vi "Calc Arc Angles.vi"(9 "Position Scale":dbl=1.0, 10 "Arc CMD":T1={"N"=0.0, "GCODE"="", "X"=2.0396, "Y"=0.1665, "Z"=0.0, "E"=0.0, "I"=0.205, "J"=0.131, "S"=0.0, "F"=0.0, "Text"=""}, 11 "Initial CMD":T1={"N"=0.0, "GCODE"="", "X"=1.6296, "Y"=0.1665, "Z"=-0.05, "E"=0.0, "I"=0.0, "J"=0.0, "S"=0.0, "F"=0.0, "Text"=""}) -> (0 "travel angle out":dbl=114.84085989051317 format="%.5f", 2 "start angle (tangent)":dbl=212.57957005474344 format="%#_8g", 3 "R":dbl=0.2432817296880306 format="%#_9g")   [LabVIEW 2014]
uses:
  GCode Parser/GCode Command Cluster.ctl
panel:
  out "x*y":dbl=32.57957005474343
  out "V2Y":dbl=-0.13099999999999998
  out "V2X":dbl=0.20500000000000007
  out "V1Y":dbl=-0.13099999999999998
  out "V1X":dbl=-0.20500000000000007
  out "theta (degrees)":dbl=-114.84085989051317 format="%.2f"
  out "theta (radians)":dbl=-2.0043511209109495 format="%.3f"
  # "G01 X1.6296 Y0.1665 Z-0.0500\nG03 X2.0396 Y0.1665 I0.2050 J0.1310"
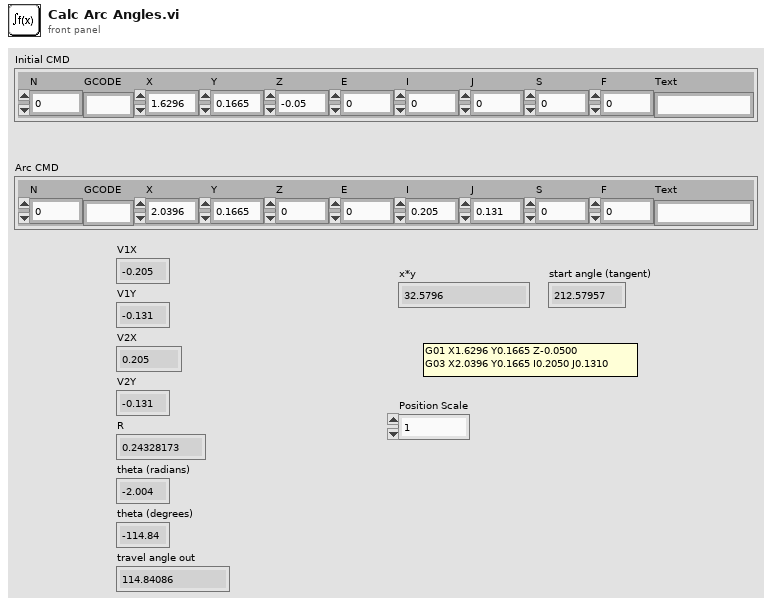
[diagram p1: front panel]
types:
  T1 = typedef "GCode Command Cluster.ctl" = cluster{"N":dbl, "GCODE":string, "X":dbl, "Y":dbl, "Z":dbl, "E":dbl, "I":dbl, "J":dbl, "S":dbl, "F":dbl, "Text":string}
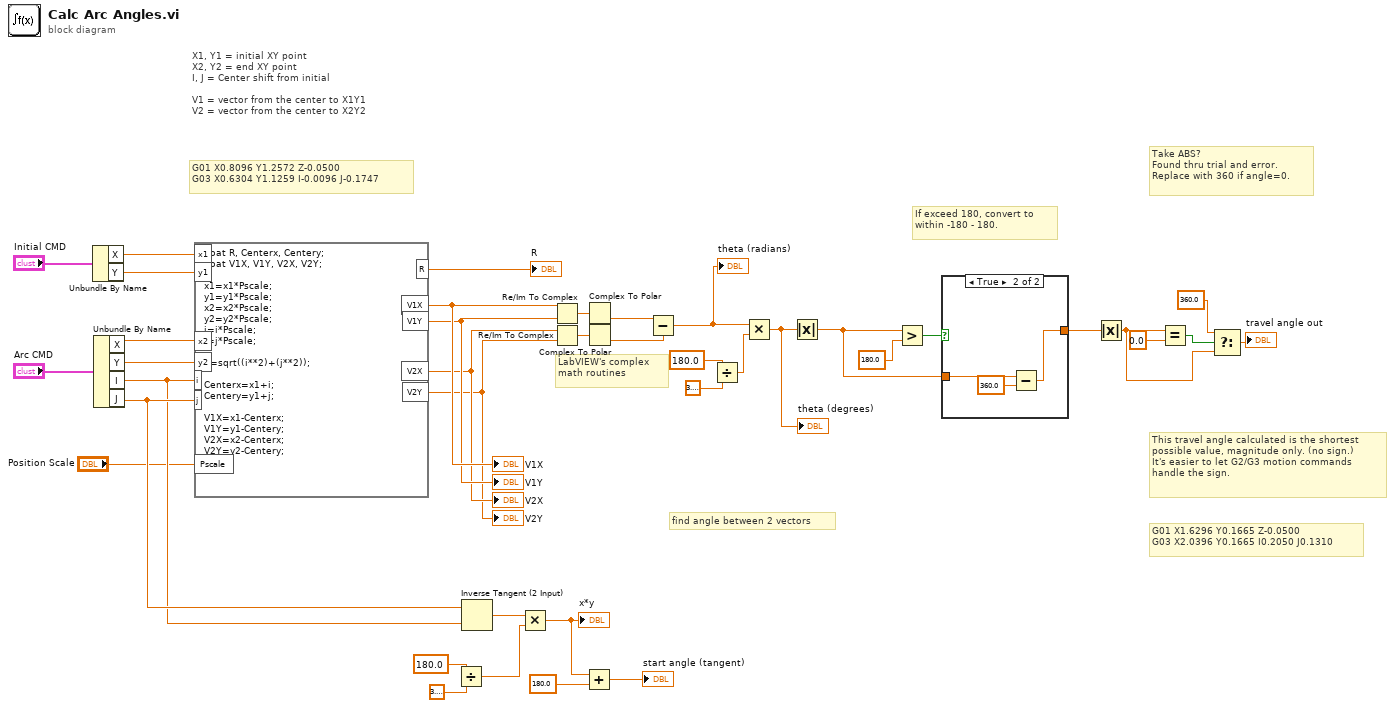
[diagram p0: block diagram]
diagram:
  # "This travel angle calculated is the shortest\npossible value, magnitude only. (no sign.)\nIt's easier to let G2/G3 motion commands\nhandle the sign."
  # "If exceed 180, convert to \nwithin -180 - 180."
  # "G01 X1.6296 Y0.1665 Z-0.0500\nG03 X2.0396 Y0.1665 I0.2050 J0.1310"
  # "Take ABS?\nFound thru trial and error.\nReplace with 360 if angle=0."
  # "find angle between 2 vectors"
  # "X1, Y1 = initial XY point\nX2, Y2 = end XY point\nI, J = Center shift from initial \n\nV1 = vector from the center to X1Y1\nV2 = vector from the center to X2Y2"
  # "LabVIEW's complex\nmath routines"
  # "G01 X0.8096 Y1.2572 Z-0.0500\nG03 X0.6304 Y1.1259 I-0.0096 J-0.1747"
  n1 = Unbundle By Name("Initial CMD") -> ("X"=w19:dbl, "Y"=w20:dbl)
  n2 = Unbundle By Name("Arc CMD") -> ("X"=w18:dbl, "Y"=w17:dbl, "I"=w15:dbl, "J"=w16:dbl)
  n3 = formula code="float R, Centerx, Centery;\nfloat V1X, V1Y, V2X, V2Y;\n\nx1=x1*Pscale;\ny1=y1*Pscale;\nx2=x2*Pscale;\ny2=y2*Pscale;\ni=i*Pscale;\nj=j*Pscale;\n\nR=sqrt((i**2)+(j**2));\n\nCenterx=x1+i;\nCentery=y1+j;\n\nV1X=x1-Centerx;\nV1Y=y1-Centery;\nV2X=x2-Centerx;\nV2Y=y2-Centery;"("x2"=w18, "x1"=w19, "y2"=w17, "y1"=w20, "i"=w15, "j"=w16, "Pscale"="Position Scale") -> ("R"=→"R":dbl, "V1X"=w30:dbl, "V1Y"=w29:dbl, "V2X"=w28:dbl, "V2Y"=w27:dbl)
  "V1X" <- w30
  "V1Y" <- w29
  "V2X" <- w28
  "V2Y" <- w27
  n4 = Divide(x=180.0, y=3.141592653589793) -> (x/y=w12:dbl)
  n5 = Inverse Tangent (2 Input)(1:w15, 2:w16) -> (0:w11:dbl)
  n6 = Multiply(x=w11, y=w12) -> (x*y=w7:dbl)
  "x*y" <- w7
  n7 = Re/Im To Complex(1:w29, 2:w30) -> (0:w38:cdb)
  n8 = Re/Im To Complex(1:w27, 2:w28) -> (0:w37:cdb)
  n9 = Add(x=w7, y=180.0) -> (x+y=→"start angle (tangent)":dbl)
  n10 = Complex To Polar(r * e^(i*theta)=w38) -> (theta=w33:dbl)  [unwired: 1 out]
  n11 = Complex To Polar(r * e^(i*theta)=w37) -> (theta=w32:dbl)  [unwired: 1 out]
  n12 = Subtract(x=w33, y=w32) -> (x-y=w34:dbl)
  "theta (radians)" <- w34
  n13 = Divide(x=180.0, y=3.141592653589793) -> (x/y=w31:dbl)
  n14 = Multiply(x=w34, y=w31) -> (x*y=w5:dbl)
  "theta (degrees)" <- w5
  n15 = Absolute Value(x=w5) -> (abs(x)=w3:dbl)
  n16 = Greater?(x=w3, y=180.0) -> (0:w2:bool)
  n17 = case shown="True" w2 {
    tunnel: w3 -> [w40 w43]
    tunnel: [w40 w41] -> w6
    frame False {
    }
    frame True {
      n18 = Subtract(x=w43, y=360.0) -> (x-y=w41:dbl)
    }
  }
  n19 = Absolute Value(x=w6) -> (abs(x)=w10:dbl)
  n20 = Equal?(x=w10, y=0.0) -> (x = y?=w26:bool)
  n21 = Select(t=360.0, s=w26, f=w10) -> (s? t:f=→"travel angle out":dbl)
